vi "PH_PSDBWriter.Wrap Boolean Data.vi"(1 "Unit Array":string[](array[string]), 2 "Data Array":bool[](array[boolean]), 3 "Name Array":string[](array[string]), 4 "Name Prefix":string) -> (0 "PSDB Boolean Data Array":T1[](array[typedef]))   [LabVIEW 2014, in "PH_PSDBWriter.lvlib"]
doc: "This VI wrapes boolean data for the PSDB."
uses:
  PH_PSDBWriter.lvlib
  PH_PSDBWriter.Boolean dataset.ctl
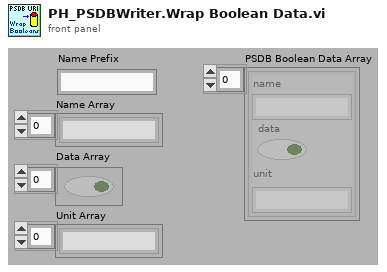
[diagram p1: front panel]
types:
  T1 = typedef "PH_PSDBWriter.lvlib/PH_PSDBWriter.Boolean dataset.ctl" = cluster{"name":string, "data":bool, "unit":string}
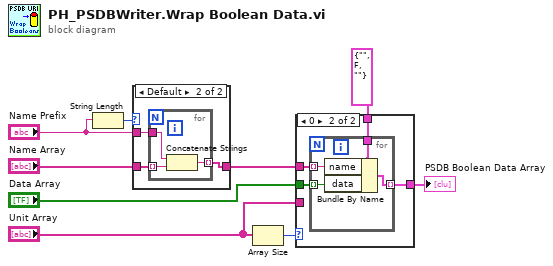
[diagram p0: block diagram]
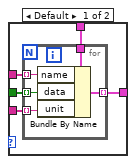
[diagram p2: hidden frame]
diagram:
  n1 = String Length(string="Name Prefix") -> (length=w5:i32)
  n2 = case shown="Default" w5 {
    tunnel: "Name Array" -> [w10 w13]
    tunnel: [w10 w11] -> w2
    tunnel: "Name Prefix" -> [_ w12]
    frame 0 {
    }
    frame Default {
      n3 = for {
        tunnel: w13 -> [w16] mode=indexing
        tunnel: w12 -> [w15]
        tunnel: [w14] -> w11 mode=indexing
        n4 = Concatenate Strings(w15, w16) -> (w14:string)
      }
    }
  }
  n5 = Array Size(array="Unit Array") -> (size(s)=w1:i32)
  n6 = case shown="0" w1 {
    tunnel: "Unit Array" -> [w21 _]
    tunnel: T1 {"name"="", "data"=FALSE, "unit"=""} ("Boolean data") -> [w20 w30]
    tunnel: "Data Array" -> [w19 w29]
    tunnel: [w18 w28] -> w6
    tunnel: w2 -> [w17 w27]
    frame Default {
      n7 = for {
        tunnel: w20 -> [w26]
        tunnel: w19 -> [w25] mode=indexing
        tunnel: w17 -> [w24] mode=indexing
        tunnel: [w23] -> w18 mode=indexing
        tunnel: w21 -> [w22] mode=indexing
        n8 = Bundle By Name(cluster=w26, "name"=w24, "data"=w25, "unit"=w22) -> (w23:T1)
      }
    }
    frame 0 {
      n9 = for {
        tunnel: w30 -> [w34]
        tunnel: w29 -> [w33] mode=indexing
        tunnel: w27 -> [w32] mode=indexing
        tunnel: [w31] -> w28 mode=indexing
        n10 = Bundle By Name(cluster=w34, "name"=w32, "data"=w33) -> (w31:T1)
      }
    }
  }
  "PSDB Boolean Data Array" <- w6
